vi "FactoryCalPopupTimeDelay.vi"(8 "error in":errorcluster, 10 "DaysToAdd":dbl) -> (0 "error out":errorcluster, 2 "TripPopUp(T)":bool)   [LabVIEW 2018]
uses:
  Initialize References/Sequence Globals.vi
panel:
  out "date/time string":string="3/1/2025 1:03:06 PM"
  out "x+y":timestamp=timestamp(3823696986.0002174 s since 1904-01-01)
  out "Date/Time From File":string="2/7/2025 5:34:11 PM"
  in  "file path(path)":path=path "C:/RageATE/Automated Tests/Tetra WAM/PRODUCTION/Test Benches/Common/CalPopupTimer.txt"
  out "current date/time(str)":string="2/11/2025 1:03:06 PM"
  out "Timestamp from Date/Time String":timestamp=timestamp(3821812451 s since 1904-01-01)
  out "current time(TS)":timestamp=timestamp(3822141786.0002174 s since 1904-01-01)
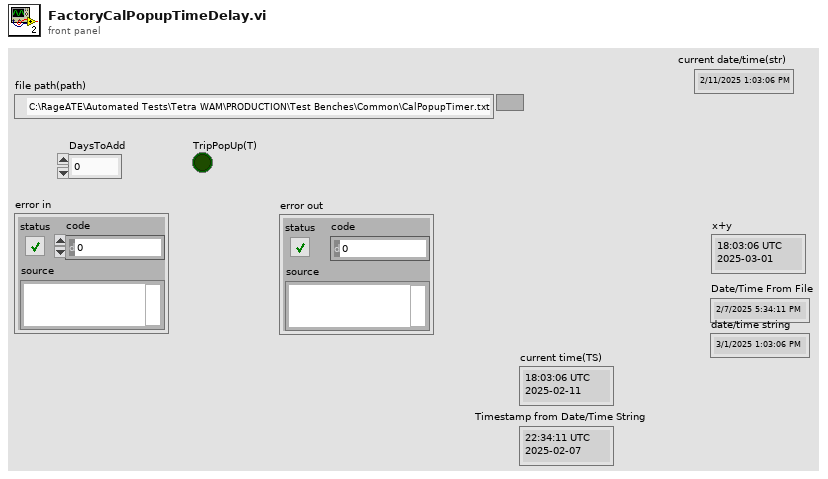
[diagram p1: front panel]
types:
  T1 = enum16{"open", "replace", "create", "open or create", "replace or create", "replace or create with confirmation"}
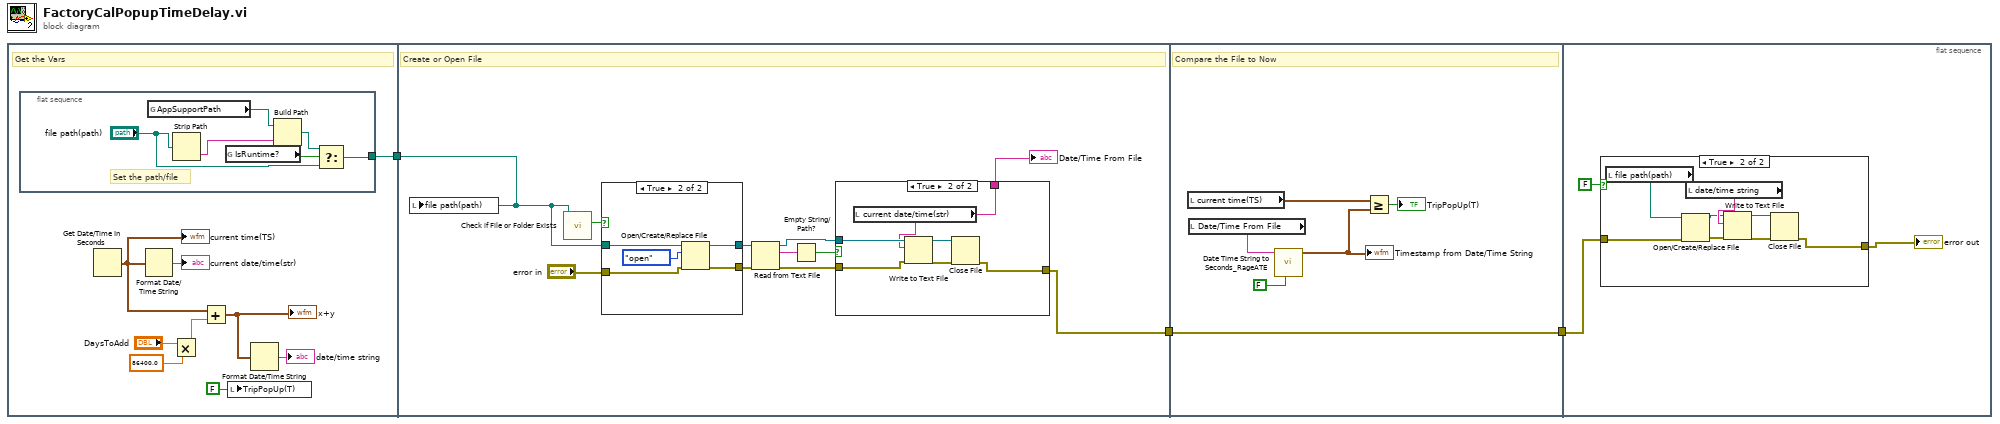
[diagram p0: block diagram]
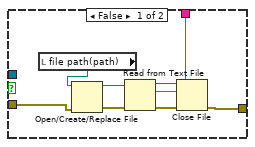
[diagram p2: hidden frame]
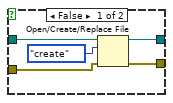
[diagram p3: hidden frame]
diagram:
  n1 = flat-sequence {
    tunnel: [w5] -> w3
    tunnel: w3 -> [w21]
    tunnel: [w20] -> w1
    tunnel: [w55] -> w2
    tunnel: w1 -> [w55]
    tunnel: w2 -> [w62]
    frame #0 {
      # "Get the Vars"
      n2 = flat-sequence {
        tunnel: [w13] -> w5
        frame #0 {
          # "Set the path/file"
          n3 = global read "Sequence Globals.vi" "AppSupportPath"() -> (w14:path)
          n4 = Strip Path(path="file path(path)") -> (name=w15:string)  [unwired: 1 out]
          n5 = global read "Sequence Globals.vi" "IsRuntime?"() -> (w17:bool)
          n6 = Build Path(base path=w14, name or relative path=w15) -> (appended path=w16:path)
          n7 = Select(t=w16, s=w17, f="file path(path)") -> (s? t:f=w13:path)
        }
      }
      n8 = Get Date/Time In Seconds() -> (seconds since 1Jan1904=w11:timestamp)
      "current time(TS)" <- w11
      n9 = Format Date/Time String(seconds (now)=w11) -> (date/time string=→"current date/time(str)":string)  [unwired: 2 in]
      n10 = Multiply(x="DaysToAdd", y=86400.0) -> (x*y=w9:dbl)
      n11 = Add(x=w11, y=w9) -> (x+y=w7:timestamp)
      "x+y" <- w7
      n12 = local write "TripPopUp(T)"(FALSE ("TripPopUp(T)")) -> ()
      n13 = Format Date/Time String(seconds (now)=w7) -> (date/time string=→"date/time string":string)  [unwired: 2 in]
    }
    frame #1 {
      # "Create or Open File"
      n14 = local write "file path(path)"(w21) -> ()
      n15 = call <vilib>:"Check if File or Folder Exists.vi"("path"=w21) -> ("file or folder exists?"=w19:bool)  [unwired: 8 in, 2 out]
      n16 = case shown="True" w19 {
        tunnel: [w48 w53] -> w24
        tunnel: w21 -> [w46 w51]
        tunnel: [w45 w50] -> w28
        tunnel: "error in" -> [w44 w49]
        frame False {
          n17 = Open/Create/Replace File(file path (use dialog)=w46, error in=w44, operation (0:open)=T1."create") -> (refnum out=w48:refnum<file>, error out=w45:errorcluster)  [unwired: 3 in, 1 out]
        }
        frame True {
          n18 = Open/Create/Replace File(file path (use dialog)=w51, error in=w49, operation (0:open)=T1."open") -> (refnum out=w53:refnum<file>, error out=w50:errorcluster)  [unwired: 3 in, 1 out]
        }
      }
      n19 = Read from Text File(file (use dialog)=w24, error in=w28) -> (refnum out=w25:refnum<file>, text=w23:string, error out=w27:errorcluster)  [unwired: 2 in, 1 out]
      n20 = Empty String/Path?(string/path=w23) -> (empty?=w26:bool)
      n21 = case shown="True" w26 {
        tunnel: w25 -> [_ w43]
        tunnel: [w30 w39] -> w20
        tunnel: w27 -> [w32 w42]
        tunnel: [w34 w40] -> w22
        frame False {
          n22 = local read "file path(path)"() -> (w33:path)
          n23 = Open/Create/Replace File(file path (use dialog)=w33, error in=w32) -> (refnum out=w35:refnum<file>, error out=w31:errorcluster)  [unwired: 4 in, 1 out]
          n24 = Read from Text File(file (use dialog)=w35, error in=w31) -> (refnum out=w37:refnum<file>, text=w34:string, error out=w36:errorcluster)  [unwired: 2 in, 1 out]
          n25 = Close File(refnum=w37, error in=w36) -> (error out=w30:errorcluster)  [unwired: 1 out]
        }
        frame True {
          n26 = local read "current date/time(str)"() -> (w40:string)
          n27 = Write to Text File(file (use dialog)=w43, text=w40, error in=w42) -> (refnum out=w41:refnum<file>, error out=w38:errorcluster)  [unwired: 1 in, 1 out]
          n28 = Close File(refnum=w41, error in=w38) -> (error out=w39:errorcluster)  [unwired: 1 out]
        }
      }
      "Date/Time From File" <- w22
    }
    frame #2 {
      # "Compare the File to Now"
      n29 = local read "current time(TS)"() -> (w57:timestamp)
      n30 = local read "Date/Time From File"() -> (w58:string)
      n31 = call "Date Time String to Seconds_RageATE.vi"("DST"=FALSE, "Time/date(str)in"=w58) -> ("Timestamp from Date/Time String"=w56:timestamp)  [unwired: 7 in, 2 out]
      "Timestamp from Date/Time String" <- w56
      n32 = Greater Or Equal?(x=w57, y=w56) -> (x >= y?=→"TripPopUp(T)":bool)
    }
    frame #3 {
      n33 = case shown="True" FALSE {
        tunnel: [w63 w69] -> w61
        tunnel: w62 -> [w63 w64]
        frame False {
        }
        frame True {
          n34 = local read "file path(path)"() -> (w66:path)
          n35 = Open/Create/Replace File(file path (use dialog)=w66, error in=w64) -> (refnum out=w67:refnum<file>, error out=w65:errorcluster)  [unwired: 4 in, 1 out]
          n36 = local read "date/time string"() -> (w70:string)
          n37 = Write to Text File(file (use dialog)=w67, text=w70, error in=w65) -> (refnum out=w71:refnum<file>, error out=w68:errorcluster)  [unwired: 1 in, 1 out]
          n38 = Close File(refnum=w71, error in=w68) -> (error out=w69:errorcluster)  [unwired: 1 out]
        }
      }
      "error out" <- w61
    }
  }
